vi "readOutcomes.vi"(8 "error in (no error)":errorcluster, 10 "WhichMonth":refnum<class "WhichMonth.lvclass">, 11 "Database in":refnum<class "Account History.lvclass">) -> (0 "error out":errorcluster, 2 "OutcomeList.lvclass":refnum<class "OutcomeList.lvclass">, 3 "Database out":refnum<class "Account History.lvclass">)   [LabVIEW 2018, in "Account History.lvclass"]
uses:
  Account History.lvclass
  WhichMonth/WhichMonth.lvclass
  OutcomeList/OutcomeList.lvclass
  Expense Summary/Outcome.lvclass
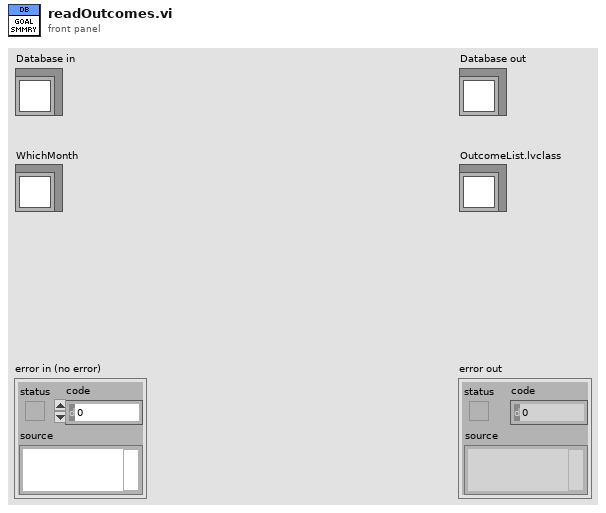
[diagram p1: front panel]
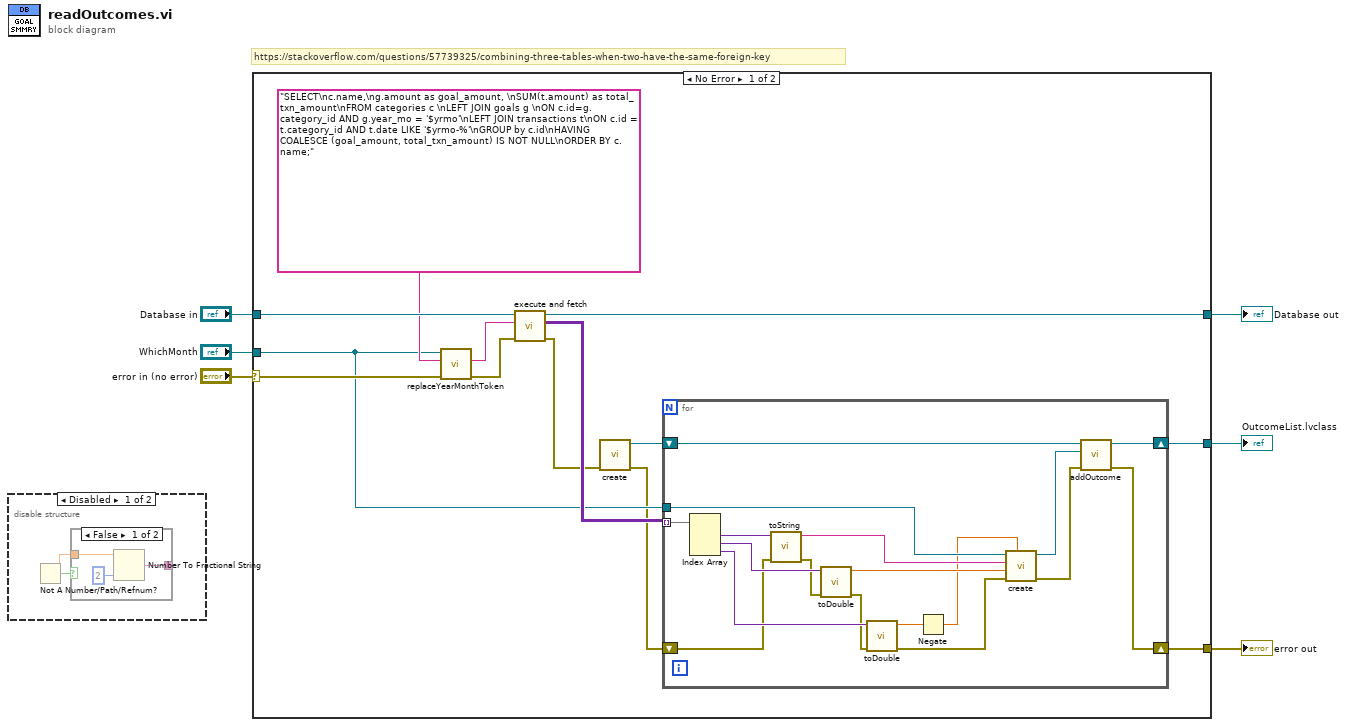
[diagram p0: block diagram]
diagram:
  # "https://stackoverflow.com/questions/57739325/combining-three-tables-when-two-have-the-same-foreign-key"
  n1 = disable-structure shown="Disabled" {
    frame Disabled {
      n2 = Not A Number/Path/Refnum?() -> (number/path/refnum=w8:dbl, NaN/Path/Refnum?=w7:bool)
      n3 = case shown="False" w7 {
        tunnel: [w11 _] -> _
        tunnel: w8 -> [w9 _]
        frame False {
          n4 = Number To Fractional String(number=w9, precision (6)=i16 2) -> (F-format string=w11:string)  [unwired: 2 in]
        }
        frame True {
        }
      }
    }
    frame Enabled {
    }
  }
  n5 = case shown="No Error" "error in (no error)" {
    selector: "error in (no error)" -> [w21 w43]
    tunnel: [w23 w44] -> w6
    tunnel: "Database in" -> [w22 w44]
    tunnel: [w17 w43] -> w4
    tunnel: "WhichMonth" -> [w16 _]
    tunnel: [w12 _] -> w1
    frame No Error {
      n6 = call "replaceYearMonthToken.vi"("error in (no error)"=w21, "Query In"="SELECT\nc.name,\ng.amount as goal_amount, \nSUM(t.amount) as total_txn_amount\nFROM categories c \nLEFT JOIN goals g \nON c.id=g.category_id AND g.year_mo = '$yrmo'\nLEFT JOIN transactions t\nON c.id = t.category_id AND t.date LIKE '$yrmo-%'\nGROUP by c.id\nHAVING COALESCE (goal_amount, total_txn_amount) IS NOT NULL\nORDER BY c.name;", "WhichMonth in"=w16) -> ("error out"=w20:errorcluster, "Query Out"=w18:string)  [unwired: 6 in, 1 out]
      n7 = call "execute and fetch.vi"("error in (no error)"=w20, "SQL query"=w18, "Database in"=w22) -> ("error out"=w15:errorcluster, "recordset data"=w24:variant[][], "Database out"=w23:refnum<class "Account History.lvclass">)  [unwired: 5 in, 1 out]
      n8 = call "create.vi"("error in (no error)"=w15) -> ("error out"=w14:errorcluster, "OutcomeList out"=w13:refnum<class "OutcomeList.lvclass">)  [unwired: 9 in]
      n9 = for {
        tunnel: w24 -> [w42] mode=indexing
        shift-right: [w25] -> w17
        shift-left: w14 -> [w38]
        tunnel: w16 -> [w34]
        shift-right: [w28] -> w12
        shift-left: w13 -> [w29]
        n10 = Index Array(array=w42) -> (element #1=w41:variant, element #2=w40:variant, element #3=w39:variant)  [unwired: 3 in]
        n11 = call "toString.vi"("error in (no error)"=w38, "Variant"=w41) -> ("error out"=w37:errorcluster, "String"=w35:string)  [unwired: 8 in]
        n12 = call "toDouble.vi"("error in (no error)"=w37, "Value"=w40) -> ("error out"=w36:errorcluster, "type"=w33:dbl)  [unwired: 8 in]
        n13 = call "toDouble.vi"("error in (no error)"=w36, "Value"=w39) -> ("error out"=w31:errorcluster, "type"=w32:dbl)  [unwired: 8 in]
        n14 = Negate(x=w32) -> (-x=w30:dbl)
        n15 = call "create.vi"("Actual"=w30, "error in (no error)"=w31, "Amount"=w33, "Category Name"=w35, "WhichMonth.lvclass"=w34) -> ("error out"=w26:errorcluster, "Outcome out"=w27:refnum<class "Outcome.lvclass">)  [unwired: 5 in]
        n16 = call "addOutcome.vi"("error in (no error)"=w26, "Outcome.lvclass"=w27, "OutcomeList in"=w29) -> ("error out"=w25:errorcluster, "OutcomeList out"=w28:refnum<class "OutcomeList.lvclass">)  [unwired: 7 in]
      }
    }
    frame Error {
    }
  }
  "error out" <- w4
  "Database out" <- w6
  "OutcomeList.lvclass" <- w1
